vi "Beamline Safety check.vi"(8 "error in":errorcluster, 9 "Current State Array":bool[](array[boolean]), 10 "Is Safe Array":bool[](array[boolean]), 11 "Task Array":refnum<k21>[](array[refnum])) -> (0 "error out":errorcluster, 1 "Task Array":refnum<k21>[](array[refnum]), 2 "Safe conditions":bool, 3 "Multiple Unsafe":bool, 5 "Index Array":i32[](array[numeric]))   [LabVIEW 2013]
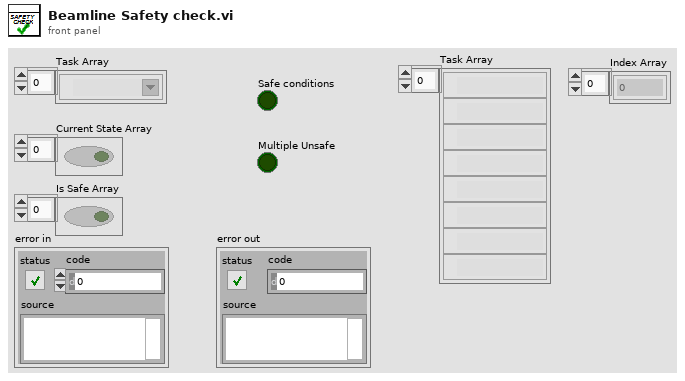
[diagram p1: front panel]
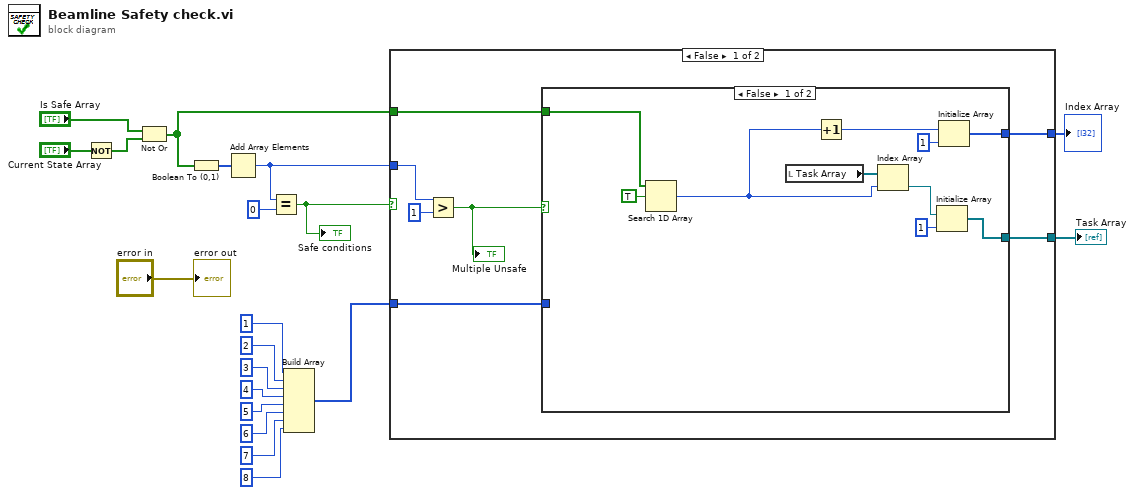
[diagram p0: block diagram]
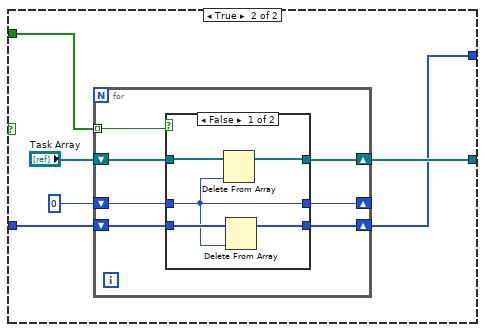
[diagram p2: hidden frame]
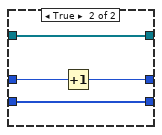
[diagram p3: hidden frame]
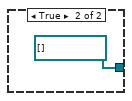
[diagram p4: hidden frame]
diagram:
  n1 = Not(x="Current State Array") -> (.not. x?=w1:bool[])
  n2 = Not Or(1:w1, 2:"Is Safe Array") -> (0:w18:bool[])
  n3 = Boolean To (0,1)(Boolean=w18) -> (0, 1=w17:i16[])
  n4 = Add Array Elements(numeric array=w17) -> (sum=w16:i16)
  n5 = Equal?(x=w16, y=u32 0) -> (x = y?=w19:bool)
  "Safe conditions" <- w19
  n6 = Build Array(1, 2, 3, 4, 5, 6, 7, 8) -> (w2:i32[])
  n7 = case shown="False" w19 {
    tunnel: w16 -> [w26 _]
    tunnel: w18 -> [w25 _]
    tunnel: [w23 refnum<k21>[] []] -> w15
    tunnel: [w22 _] -> w11
    tunnel: w2 -> [w21 _]
    frame False {
      n8 = Greater?(x=w26, y=u32 1) -> (0:w24:bool)
      "Multiple Unsafe" <- w24
      n9 = case shown="False" w24 {
        tunnel: w25 -> [w36 w43]
        tunnel: [w33 w42] -> w23
        tunnel: [w30 w39] -> w22
        tunnel: w21 -> [_ w38]
        frame False {
          n10 = Search 1D Array(1D array=w36, element=TRUE) -> (index of element=w31:i32)  [unwired: 1 in]
          n11 = local read "Task Array"() -> (w37:refnum<k21>[])
          n12 = Increment(x=w31) -> (x+1=w28:i32)
          n13 = Index Array(array=w37, index=w31) -> (element=w34:refnum<k21>)
          n14 = Initialize Array(w34, 1 ("dimension size")) -> (w33:refnum<k21>[])
          n15 = Initialize Array(w28, 1 ("dimension size")) -> (w30:i32[])
        }
        frame True {
          n16 = for {
            tunnel: w43 -> [w50] mode=indexing
            shift-right: [w48] -> w42
            shift-left: "Task Array" -> [w49]
            shift-right: [w46] -> _
            shift-left: 0 -> [w47]
            shift-right: [w45] -> w39
            shift-left: w38 -> [w44]
            n17 = case shown="False" w50 {
              tunnel: w49 -> [w55 w59]
              tunnel: [w54 w59] -> w48
              tunnel: w47 -> [w52 w58]
              tunnel: [w52 w57] -> w46
              tunnel: [w51 w56] -> w45
              tunnel: w44 -> [w53 w56]
              frame False {
                n18 = Delete From Array(array=w55, index=w52) -> (array with subset deleted=w54:refnum<k21>[])  [unwired: 1 in, 1 out]
                n19 = Delete From Array(array=w53, index=w52) -> (array with subset deleted=w51:i32[])  [unwired: 1 in, 1 out]
              }
              frame True {
                n20 = Increment(x=w58) -> (x+1=w57:i32)
              }
            }
          }
        }
      }
    }
    frame True {
    }
  }
  "Task Array" <- w15
  "Index Array" <- w11
  "error out" <- "error in"
